vi "Data Viewer.vi"(6 "menu options":cluster{"open":bool, "save":bool, "view":bool}={"open"=TRUE, "save"=FALSE, "view"=FALSE}, 8 "error in (no error)":errorcluster, 9 "Stop Pointer":refnum<class "Pointer.lvclass">, 10 "Framework Configuration":T1, 11 "DSF":refnum<class "Framework.lvclass">) -> (0 "error out":errorcluster)   [LabVIEW 2017, in "DSF Core.lvlib"]
uses:
  DSF Core.lvlib
  Classes/Framework/Framework.lvclass
  Typedefs/DSF Engine Framework Configuration.ctl
  Typedefs/DSF Engine Plugin Configuration.ctl
  Typedefs/DSF Timing Info.ctl
  Typedefs/DSF Engine Plugin Thread Configuration.ctl
  Typedefs/DSF Settings Info.ctl
  Typedefs/DSF Engine Transfer Group Configuration.ctl
  Typedefs/DSF Direction.ctl
  Typedefs/DSF Engine Transfer Configuration.ctl
  Typedefs/DSF Byte Order.ctl
  Typedefs/DSF Engine Channel Configuration.ctl
  Typedefs/DSF Data Type.ctl
  Typedefs/DSF Timeout Behavior.ctl
  <vilib>/NI/Memory Manager/Classes/Pointer/Pointer.lvclass
  <vilib>/NI/Memory Manager/Classes/Pointer/Pointer.lvclass/Pointer.ctl
  Classes/Framework/Framework.lvclass/Framework.ctl
  Source/Main VI/Application Data.ctl
  Source/Buffer Reader/Buffer Data.ctl
  Classes/Buffer/Buffer.lvclass
  C:/Program Files (x86)/National Instruments/LabVIEW 2017/vi.lib/NI/Memory Manager/Classes/Pointer/Pointer.lvclass
  Classes/Transfer Group Status/Status.lvclass
  Classes/Performance/Performance.lvclass/Performance.ctl
  <vilib>/NI/Memory Manager/Classes/Pointer/Read Bool.vi
  <vilib>/NI/Memory Manager/Classes/Pointer/Write Bool.vi
  <vilib>/NI/Memory Manager/Classes/Pointer/Read (No Check).vi
  <vilib>/NI/Memory Manager/Classes/Pointer/Read (No Check) Bool.vi
  <vilib>/NI/Memory Manager/Classes/Pointer/Check Move.vi
  <vilib>/NI/Memory Manager/Classes/Pointer/Write (No Check).vi
  <vilib>/NI/Memory Manager/Classes/Pointer/Write (No Check) Bool.vi
  Source/Item Tree/Get Buffer Data from Variant.vi
  <vilib>/NI/Memory Manager/Classes/Pointer/Get Size.vi
  Classes/Performance/Read Timing Status.vi
  <vilib>/NI/Memory Manager/Classes/Pointer/Check Size (0D).vi
  <vilib>/NI/Memory Manager/Classes/Pointer/Get Address.vi
  Classes/Transfer Group Status/Status Size.vi
  <vilib>/NI/Memory Manager/Classes/Pointer/Check Null Pointer.vi
  <vilib>/NI/Memory Manager/Classes/Pointer/Set Address.vi
  <vilib>/NI/Memory Manager/Classes/Pointer/Set Size.vi
  <vilib>/NI/Memory Manager/Classes/Pointer/Set Internal.vi
  <vilib>/NI/Memory Manager/Classes/Pointer/Check Count.vi
  <vilib>/NI/Memory Manager/Classes/Pointer/Check Bounds (Power of 2).vi
  Classes/Timing Status/Read Timing Status.vi
  <vilib>/NI/Memory Manager/Classes/Pointer/Errors.vi
  <vilib>/NI/Memory Manager/Classes/Pointer/Out of Bounds.vi
  <vilib>/NI/Memory Manager/Classes/Pointer/Null Pointer.vi
  <vilib>/NI/Memory Manager/Classes/Pointer/Check Bounds.vi
  Classes/Timing Status/Timing Status Size.vi
  <vilib>/NI/Memory Manager/VIs/Source.Write.String.vi
  <vilib>/NI/Memory Manager/Classes/Pointer/Write Pointer Size.vi
  <vilib>/NI/Memory Manager/Classes/Pointer/Create Error.vi
  <vilib>/NI/Memory Manager/VIs/Source.Write.Scalar.Base10.vi
  <vilib>/NI/Memory Manager/VIs/Source.Write.Scalar.Base10 (U64).vi
  <vilib>/NI/Memory Manager/Classes/Pointer/Check Pointer Bounds.vi
  <vilib>/NI/Memory Manager/Classes/Pointer/Check Buffer Bounds.vi
  <vilib>/NI/Memory Manager/VIs/New Error Cluster Constant.vi
  <vilib>/NI/Memory Manager/VIs/New Error Cluster Constant (512B).vi
  <vilib>/NI/Memory Manager/VIs/Error Cluster.Set Status.vi
  <vilib>/NI/Memory Manager/VIs/Error Cluster.Set Code.vi
  <vilib>/NI/Memory Manager/VIs/Error Cluster.Set VI Source.vi
  <vilib>/NI/Memory Manager/Constants/Constants.vi
  <vilib>/NI/Memory Manager/Constants/Library Name.vi
  <vilib>/NI/Memory Manager/Classes/Pointer/Pointer Error Info.vi
  <vilib>/NI/Memory Manager/Constants/Pointer Class Name.vi
  <vilib>/NI/Memory Manager/Classes/Pointer/Buffer Underflow.vi
  Classes/Timing Status/Timing Status.lvclass
  Classes/Configuration/Required Buffer Size (Framework).vi
  Classes/Performance/Performance.lvclass
panel:
  in  "Item Tree":string(tree)
  out "Value":string
  out "Late Count":u64
  out "Iteration":u64
  out "Frequency":dbl format="%.1fHz"
  out "Size":u64 format="%#_3pB"
  out "Null Buffer":bool
  out "Decimation":u64
  out "Throughput":dbl format="%_3pB/s"
  out "Buffer":string
  # "Data Viewer"
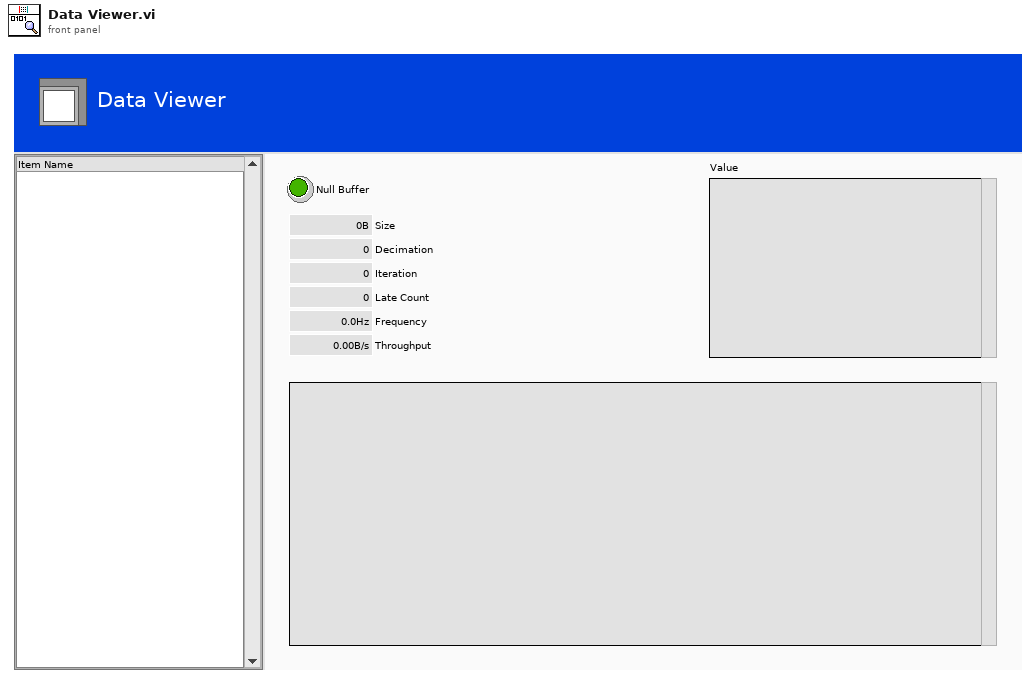
[diagram p1: front panel]
types:
  T1 = typedef "DSF Core.lvlib/DSF Engine Framework Configuration.ctl" = cluster{"components directory":path, "Plugins":T2[]}
  T2 = typedef "DSF Core.lvlib/DSF Engine Plugin Configuration.ctl" = cluster{"name":string, "components":string[], "cycle timing":T3, "threads":T4[], "Transfer Groups":T6[], "settings":T5}
  T3 = typedef "DSF Core.lvlib/DSF Timing Info.ctl" = cluster{"priority":u64, "decimation":u64, "offset":u64}
  T4 = typedef "DSF Core.lvlib/DSF Engine Plugin Thread Configuration.ctl" = cluster{"buffer converter settings":T5, "transceiver settings":T5, "processor":i32, "priority offset":i16}
  T5 = typedef "DSF Core.lvlib/DSF Settings Info.ctl" = cluster{"key":string, "value":string}[]
  T6 = typedef "DSF Core.lvlib/DSF Engine Transfer Group Configuration.ctl" = cluster{"name":string, "direction":T7, "cycle timing":T3, "thread index":i32, "settings":T5, "Transfers":T8[], "timeout behavior":T12}
  T7 = typedef "DSF Core.lvlib/DSF Direction.ctl" = enum8{"Tx", "Rx"}
  T8 = typedef "DSF Core.lvlib/DSF Engine Transfer Configuration.ctl" = cluster{"name":string, "byte order":T9, "settings":T5, "channels":T10[]}
  T9 = typedef "DSF Core.lvlib/DSF Byte Order.ctl" = enum8{"big-endian", "little-endian"}
  T10 = typedef "DSF Core.lvlib/DSF Engine Channel Configuration.ctl" = cluster{"string offset":u64, "string data type":T11, "engine data type":T11, "name":string, "settings":T5}
  T11 = typedef "DSF Core.lvlib/DSF Data Type.ctl" = enum8{"Bool", "SGL", "DBL", "I8", "I16", "I32", "I64", "U8", "U16", "U32", "U64"}
  T12 = typedef "DSF Core.lvlib/DSF Timeout Behavior.ctl" = enum8{"Increment Late Count", "Throw Error"}
  T13 = typedef "DSF Core.lvlib/Buffer Data.ctl" = cluster{"Buffer":refnum<class "Buffer.lvclass">, "Status":refnum<class "Status.lvclass">, "decimation":u64, "avg bandwidth":dbl}
  T14 = typedef "DSF Core.lvlib/Application Data.ctl" = cluster{"Item Tree Control":refnum<vi>, "Top-Level VI":refnum<vi>, "menu reference":refnum<k9>, "Framework":refnum<class "Framework.lvclass">, "buffer queue":refnum<queue>, "Stop Pointer":refnum<class "Pointer.lvclass">, "Buffer Variant":variant, "Framework Configuration":T1}
  T15 = typedef "DSF Core.lvlib/Status.lvclass/Status Data.ctl" = cluster{"late count":u64, "iteration":u64, "duration":u32}
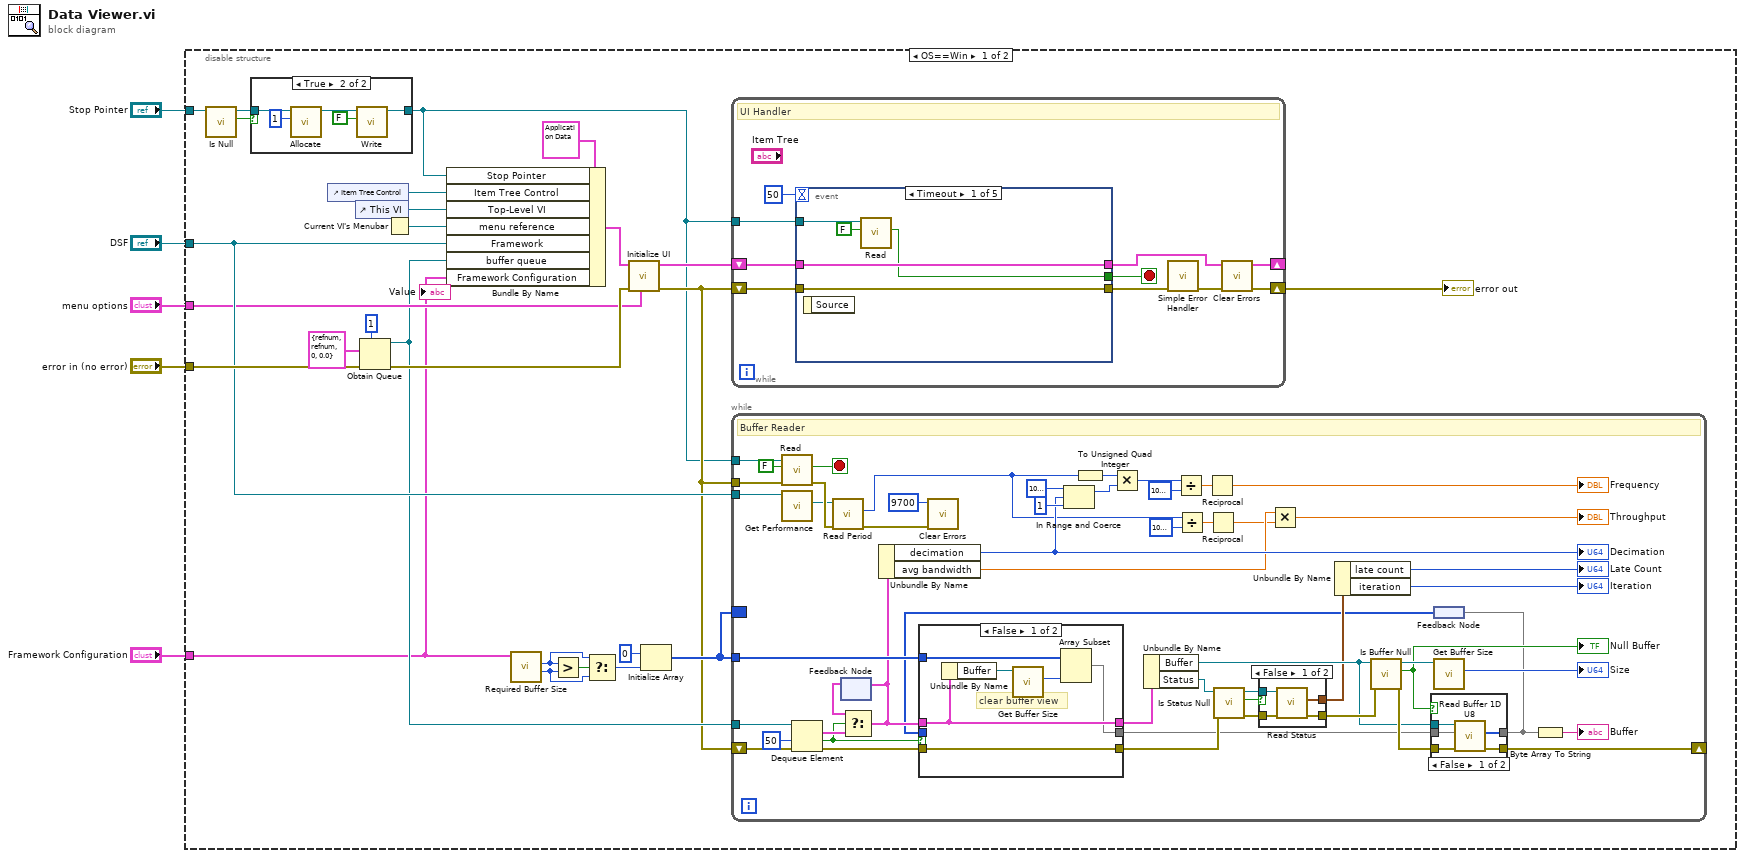
[diagram p0: block diagram]
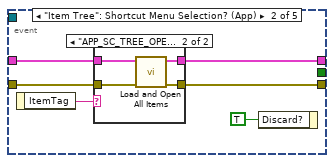
[diagram p6: hidden frame]
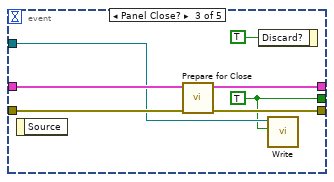
[diagram p8: hidden frame]
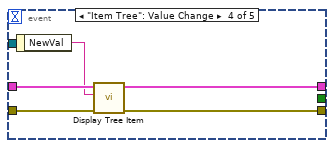
[diagram p9: hidden frame]
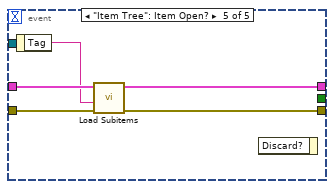
[diagram p10: hidden frame]
diagram:
  n1 = disable-structure shown="OS==Win" {
    disable-tunnel: "error in (no error)" -> [w24 _]
    disable-tunnel: "Stop Pointer" -> [w17 _]
    disable-tunnel: "DSF" -> [w15 _]
    disable-tunnel: "menu options" -> [w11 _]
    disable-tunnel: "Framework Configuration" -> [w8 _]
    frame condition #0 (active) {
      n2 = call <vilib>:"Is Null.vi"("Pointer in"=w17) -> ("null?"=w16:bool)  [unwired: 8 in, 2 out]
      n3 = case shown="True" w16 {
        tunnel: [w31 w33] -> w6
        tunnel: w17 -> [w31 w35]
        frame False {
        }
        frame True {
          n4 = call <vilib>:"Allocate.vi"("size"=u64 1, "Pointer in"=w35) -> ("Pointer out"=w34:refnum<class "Pointer.lvclass">)  [unwired: 8 in, 1 out]
          n5 = call-poly <vilib>:"Write.vi"("value"=FALSE ("buffer in"), "Pointer in"=w34) -> ("Pointer out"=w33:refnum<class "Pointer.lvclass">)  [unwired: 6 in, 3 out]
        }
      }
      n6 = control-ref of="Item Tree Control"() -> (w26:refnum<vi>)
      n7 = control-ref of="This VI"() -> (w29:refnum<vi>)
      n8 = Obtain Queue(max queue size (-1, unlimited)=1, element data type=T13 {"Buffer"=refnum, "Status"=refnum, "decimation"=0, "avg bandwidth"=0.0} ("Buffer data"), error in (no error)=w24) -> (queue out=w10:refnum<queue>, error out=w23:errorcluster)  [unwired: 2 in, 1 out]
      n9 = Current VI's Menubar() -> (w27:refnum<k9>)
      n10 = Bundle By Name(cluster=T14 {"Item Tree Control"=refnum, "Top-Level VI"=refnum, "menu reference"=refnum, "Framework"=refnum, "buffer queue"=refnum, "Stop Pointer"=refnum, "Buffer Variant"=variant, "Framework Configuration"={"components directory"=path "", "Plugins"=[]}}, "Stop Pointer"=w6, "Item Tree Control"=w26, "Top-Level VI"=w29, "menu reference"=w27, "Framework"=w15, "buffer queue"=w10, "Framework Configuration"=w8) -> (w9:T14)
      n11 = call-poly "Required Buffer Size.vi"("Framework Configuration in"=w8) -> ("total engine buffer size"=w12:u64, "total string buffer size"=w13:u64)  [unwired: 7 in, 2 out]
      n12 = Greater?(x=w13, y=w12) -> (0:w22:bool)
      n13 = Select(t=w13, s=w22, f=w12) -> (s? t:f=w20:u64)
      n14 = call "Initialize UI.vi"("menu options"=w11, "error in (no error)"=w23, "Application Data in"=w9) -> ("error out"=w7:errorcluster, "Application Data out"=w19:T14)  [unwired: 7 in]
      n15 = Initialize Array(u8 0 ("element"), w20) -> (w14:u8[])
      n16 = while {
        shift-right: [w115] -> w28
        shift-left: w7 -> [w119]
        shift-right: [w116] -> _
        shift-left: w19 -> [w114]
        tunnel: w6 -> [w112]
        stop <- w113 stop-if-true
        # "UI Handler"
        n17 = event shown="[0] Timeout" {
          selector: _ -> [_ _ _ _ _]
          dyn-events: _ -> [_ _ _ _ _]
          timeout: 50 -> [_ _ _ _ _]
          tunnel: [w120 _ w137 _ _] -> w113
          tunnel: w119 -> [w124 w127 w143 w148 w153]
          tunnel: [w124 w128 w141 w147 w152] -> w117
          tunnel: w114 -> [w123 w129 w139 w145 w151]
          tunnel: [w123 w125 w140 w146 w150] -> w116
          tunnel: w112 -> [w122 _ w138 _ _]
          event Timeout {
            n18 = event-data() -> ()  [unwired: 1 in, 1 out]
            n19 = call-poly <vilib>:"Read.vi"("value in"=FALSE ("buffer in"), "Pointer in"=w122) -> ("value out"=w120:bool)  [unwired: 6 in, 3 out]
          }
          event "Item Tree": Shortcut Menu Selection? (App) {
            n20 = event-data() -> ("ItemTag"=w130:string)  [unwired: 1 in]
            n21 = case shown="\"APP_SC_TREE_OPEN_ALL_ITEMS\"" w130 {
              tunnel: w129 -> [w131 w136]
              tunnel: [w132 w134] -> w128
              tunnel: w127 -> [w132 w135]
              tunnel: [w131 w133] -> w125
              frame Default {
              }
              frame "APP_SC_TREE_OPEN_ALL_ITEMS" {
                n22 = call "Load and Open All Items.vi"("error in (no error)"=w135, "Application Data in"=w136) -> ("error out"=w134:errorcluster, "Application Data out"=w133:T14)  [unwired: 8 in]
              }
            }
            n23 = event-data("Discard?"=TRUE) -> ()  [unwired: 1 in, 1 out]
          }
          event Panel Close? {
            w137 = TRUE
            n24 = event-data() -> ()  [unwired: 1 in, 1 out]
            n25 = call "Prepare for Close.vi"("error in (no error)"=w143, "Application Data in"=w139) -> ("error out"=w141:errorcluster, "Application Data out"=w140:T14)  [unwired: 8 in]
            n26 = event-data("Discard?"=TRUE) -> ()  [unwired: 1 in, 1 out]
            n27 = call-poly <vilib>:"Write.vi"("value"=w137, "Pointer in"=w138) -> ()  [unwired: 6 in, 4 out]
          }
          event "Item Tree": Value Change {
            n28 = event-data() -> ("NewVal"=w144:string)  [unwired: 1 in]
            n29 = call "Display Tree Item.vi"("error in (no error)"=w148, "Tag"=w144, "Application Data in"=w145) -> ("error out"=w147:errorcluster, "Application Data out"=w146:T14)  [unwired: 7 in]
          }
          event "Item Tree": Item Open? {
            n30 = event-data() -> ("Tag"=w149:string)  [unwired: 1 in]
            n31 = call "Load Subitems.vi"("error in (no error)"=w153, "Tag"=w149, "Application Data in"=w151) -> ("error out"=w152:errorcluster, "Application Data out"=w150:T14)  [unwired: 6 in, 1 out]
            n32 = event-data() -> ()  [unwired: 2 in, 1 out]
          }
        }
        n33 = call <vilib>:"Simple Error Handler.vi"("error in (no error)"=w117) -> ("error out"=w118:errorcluster)  [unwired: 4 in, 4 out]
        n34 = call <vilib>:"Clear Errors.vi"("error in (no error)"=w118) -> ("error out"=w115:errorcluster)  [unwired: 5 in, 1 out]
      }
      "error out" <- w28
      n35 = while {
        tunnel: w10 -> [w88]
        shift-right: [w67] -> _
        shift-left: w7 -> [w85]
        tunnel: w14 -> [w76]
        tunnel: w6 -> [w80]
        tunnel: w15 -> [w48]
        border: w14 -> [_]
        tunnel: w7 -> [w39]
        stop <- w81 stop-if-true
        # "Buffer Reader"
        n36 = call-poly <vilib>:"Read.vi"("error in (no error)"=w39, "value in"=FALSE ("buffer in"), "Pointer in"=w80) -> ("error out"=w38:errorcluster, "value out"=w81:bool)  [unwired: 5 in, 2 out]
        n37 = call "Get Performance.vi"("Framework in"=w48) -> ("Performance"=w37:refnum<class "Performance.lvclass">)  [unwired: 9 in, 1 out]
        n38 = Dequeue Element(queue=w88, timeout in ms (-1)=50, error in (no error)=w85) -> (element=w86:T13, timed out?=w77:bool, error out=w89:errorcluster)  [unwired: 1 out]
        n39 = call "Read Period.vi"("error in (no error)"=w38, "Framework Performance in"=w37) -> ("error out"=w68:errorcluster, "period"=w42:u32)  [unwired: 7 in, 1 out]
        n40 = feedback #1() -> (w75:T13)  [unwired: 1 in]
        n41 = Select(t=w75, s=w77, f=w86) -> (s? t:f=w71:T13)
        n42 = feedback-in #1(w71) -> ()
        n43 = Unbundle By Name(w71) -> ("decimation"=w46:u64, "avg bandwidth"=w41:dbl)
        "Decimation" <- w46
        n44 = call <vilib>:"Clear Errors.vi"("error in (no error)"=w68, "specific error code to clear (0: all)"=9700) -> ()  [unwired: 4 in, 2 out]
        n45 = In Range and Coerce(upper limit=u64 1000000000, x=w46, lower limit=u64 1) -> (coerced(x)=w45:u64)  [unwired: 1 out]
        n46 = To Unsigned Quad Integer(1:w42) -> (0:w73:u64)
        n47 = Multiply(x=w73, y=w45) -> (x*y=w84:u64)
        n48 = Divide(x=w84, y=u64 1000000) -> (x/y=w72:dbl)
        n49 = Divide(x=w42, y=u64 1000000) -> (x/y=w43:dbl)
        n50 = Reciprocal(x=w72) -> (1/x=→"Frequency":dbl)
        n51 = Reciprocal(x=w43) -> (1/x=w40:dbl)
        n52 = Multiply(x=w41, y=w40) -> (x*y=→"Throughput":dbl)
        n53 = feedback #2() -> (w50:u8[])
        n54 = case shown="False" w77 {
          tunnel: w50 -> [_ w110]
          tunnel: w71 -> [w103 w109]
          tunnel: w76 -> [w107 _]
          tunnel: [w102 w110] -> w51
          tunnel: w89 -> [w104 w108]
          tunnel: [w103 w109] -> w74
          tunnel: [w104 w108] -> w58
          frame False {
            # "clear buffer view"
            n55 = Unbundle By Name(w103) -> ("Buffer"=w105:refnum<class "Buffer.lvclass">)
            n56 = call "Get Buffer Size.vi"("Buffer in"=w105) -> ("buffer size"=w106:u64)  [unwired: 9 in, 1 out]
            n57 = Array Subset(array=w107, length=w106) -> (w102:u8[])  [unwired: 1 in]
          }
          frame True {
          }
        }
        n58 = Unbundle By Name(w74) -> ("Buffer"=w62:refnum<class "Buffer.lvclass">, "Status"=w61:refnum<class "Status.lvclass">)
        n59 = call "Is Status Null.vi"("error in (no error)"=w58, "status pointer in"=w61) -> ("error out"=w59:errorcluster, "null?"=w57:bool, "status pointer out"=w60:refnum<class "Status.lvclass">)  [unwired: 7 in]
        n60 = case shown="False" w57 {
          tunnel: [w93 w94] -> w63
          tunnel: w60 -> [w92 _]
          tunnel: w59 -> [w91 w94]
          tunnel: [w90 _] -> w56
          frame False {
            n61 = call "Read Status.vi"("error in (no error)"=w91, "status pointer in"=w92) -> ("error out"=w93:errorcluster, "status"=w90:T15)  [unwired: 7 in, 1 out]
          }
          frame True {
          }
        }
        n62 = Unbundle By Name(w56) -> ("late count"=→"Late Count":u64, "iteration"=→"Iteration":u64)
        n63 = call "Is Buffer Null.vi"("error in (no error)"=w63, "Buffer in"=w62) -> ("error out"=w65:errorcluster, "null?"=w64:bool, "Buffer out"=w66:refnum<class "Buffer.lvclass">)  [unwired: 7 in]
        "Null Buffer" <- w64
        n64 = case shown="False" w64 {
          tunnel: w65 -> [w99 w100]
          tunnel: w51 -> [w98 w101]
          tunnel: w62 -> [w97 _]
          tunnel: [w96 w101] -> w53
          tunnel: [w95 w100] -> w67
          frame False {
            n65 = call "Read Buffer 1D U8.vi"("error in (no error)"=w99, "dst array in"=w98, "Buffer in"=w97) -> ("error out"=w95:errorcluster, "dst array out"=w96:u8[])  [unwired: 5 in, 2 out]
          }
          frame True {
          }
        }
        n66 = feedback-in #2(w53) -> ()
        n67 = call "Get Buffer Size.vi"("Buffer in"=w66) -> ("buffer size"=→"Size":u64)  [unwired: 9 in, 1 out]
        n68 = Byte Array To String(unsigned byte array=w53) -> (string=→"Buffer":string)
      }
    }
    frame condition #1 {
    }
  }
